vi "AIT 429 - Add Data Channel.vi"(8 "error in (no error)":errorcluster, 11 "Node Ptr":u64 format="%.0x") -> (0 "error out":errorcluster)   [LabVIEW 2012, in "AIT 429 System Explorer.lvlib"]
uses:
  AIT 429 System Explorer.lvlib
  <vilib>/NI Veristand/Custom Device API/Custom Device Channel.ctl
  <vilib>/NI Veristand/Custom Device API/Custom Device Channel Type.ctl
  Shared/Controls and Global/Global.vi
  <vilib>/NI Veristand/Custom Device API/Get Item Property (U32).vi
  ARINC 429 Shared.lvlib
  <vilib>/NI Veristand/Custom Device API/Custom Device API.lvlib
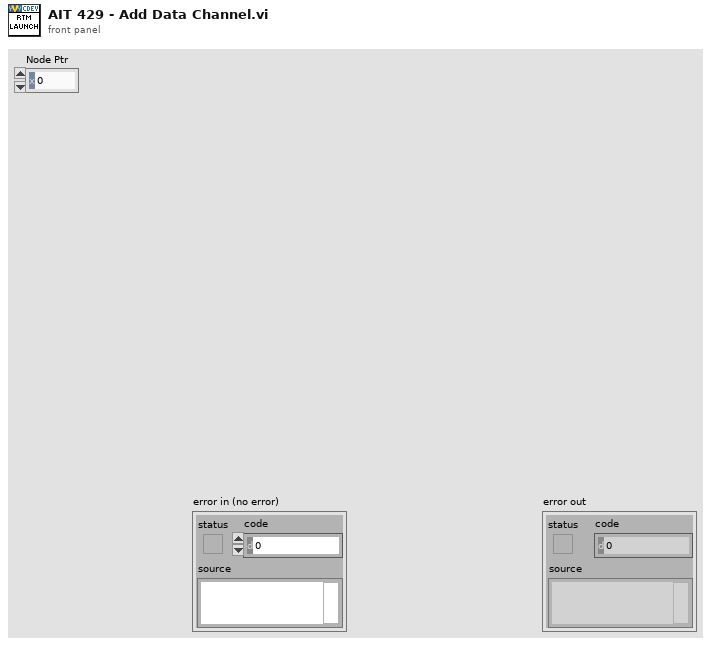
[diagram p1: front panel]
types:
  T1 = typedef "Custom Device API.lvlib/Custom Device Channel Type.ctl" = enum16{"Input", "Output"}
  T2 = typedef "Custom Device API.lvlib/Custom Device Channel.ctl" = cluster{"Type":T1, "Units":string, "Default Value":dbl, "Faultable":bool, "Scalable":bool}
  T3 = typedef "Custom Device API.lvlib/Custom Device Item Ref.ctl" = u64
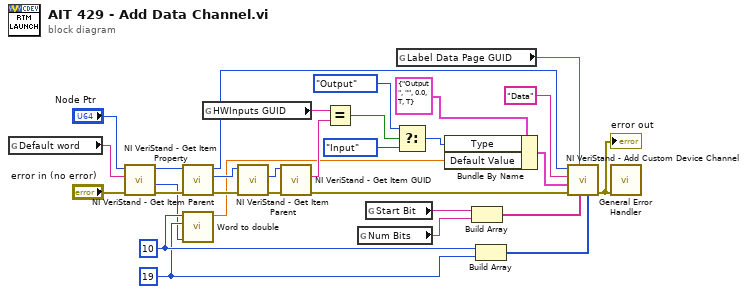
[diagram p0: block diagram]
diagram:
  w7 = 19
  w8 = 10
  n1 = global read "Global.vi" "Default word"() -> (w2:string)
  n2 = call-poly <vilib>:"NI VeriStand - Get Item Property.vi"("error in (no error)"="error in (no error)", "Property Name"=w2, "Item Ref in"="Node Ptr") -> ("error out"=w4:errorcluster, "Value"=w1:u32, "Item Ref out"=w5:T3)  [unwired: 5 in, 1 out]
  n3 = call <vilib>:"NI VeriStand - Get Item Parent.vi"("error in (no error)"=w4, "Item Ref in"=w5) -> ("error out"=w28:errorcluster, "Parent Ref"=w25:T3, "Item Ref out"=w18:T3)  [unwired: 6 in, 1 out]
  n4 = call "Word to double.vi"("word"=w1, "Number of Bits"=w7, "Start Bit"=w8) -> ("Double"=w9:dbl)  [unwired: 8 in]
  n5 = global read "Global.vi" "HWInputs GUID"() -> (w20:string)
  n6 = call <vilib>:"NI VeriStand - Get Item Parent.vi"("error in (no error)"=w28, "Item Ref in"=w25) -> ("error out"=w27:errorcluster, "Parent Ref"=w26:T3)  [unwired: 6 in, 2 out]
  n7 = call <vilib>:"NI VeriStand - Get Item GUID.vi"("error in (no error)"=w27, "Item Ref in"=w26) -> ("error out"=w13:errorcluster, "GUID"=w19:string)  [unwired: 7 in, 1 out]
  n8 = Equal?(x=w20, y=w19) -> (x = y?=w15:bool)
  n9 = global read "Global.vi" "Num Bits"() -> (w30:string)
  n10 = global read "Global.vi" "Start Bit"() -> (w16:string)
  n11 = global read "Global.vi" "Label Data Page GUID"() -> (w29:string)
  n12 = Select(t=Custom_Device_Channel_Type."Output" ("Type"), s=w15, f=Custom_Device_Channel_Type."Input" ("Type")) -> (s? t:f=w23:T1)
  n13 = Bundle By Name(cluster=T2 {"Type"=enum."Output", "Units"="", "Default Value"=0.0, "Faultable"=TRUE, "Scalable"=TRUE} ("Channel"), "Type"=w23, "Default Value"=w9) -> (w11:T2)
  n14 = Build Array(w16, w30) -> (w17:string[])
  n15 = Build Array(w8, w7) -> (w12:i32[])
  n16 = call <vilib>:"NI VeriStand - Add Custom Device Channel.vi"("Property Values"=w12, "Property names"=w17, "GUID (Default Channel)"=w29, "error in (no error)"=w13, "Channel"=w11, "Channel Name"="Data", "Parent Ref in"=w18) -> ("error out"=w14:errorcluster)  [unwired: 1 in, 3 out]
  "error out" <- w14
  n17 = call <vilib>:"General Error Handler.vi"("error in (no error)"=w14) -> ()  [unwired: 10 in, 5 out]
